vi "Turn On Change Flag Upstream.vi"(8 "symbol to change":T2, 9 "refresh listbox":T1[](array[typedef])) -> (1 "refresh listbox out":T1[](array[typedef]))   [LabVIEW 2020, in "AIM ARINC 429 System Explorer.lvlib" / "Implementation.lvlib"]
uses:
  Implementation.lvlib
  Types/Refresh Symbols.ctl
  Types/Refresh Listbox.ctl
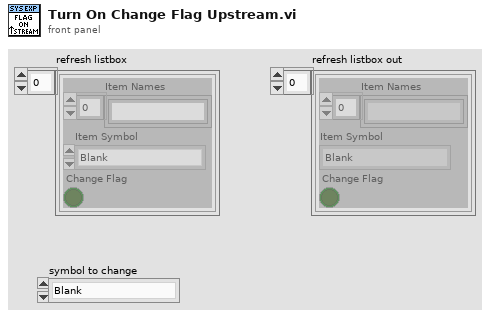
[diagram p1: front panel]
types:
  T1 = typedef "AIM ARINC 429 System Explorer.lvlib/Implementation.lvlib/Refresh Listbox.ctl" = cluster{"Item Names":string[], "Item Symbol":T2, "Change Flag":bool}
  T2 = typedef "AIM ARINC 429 System Explorer.lvlib/Implementation.lvlib/Refresh Symbols.ctl" = enum16{"Blank", "Port", "Incoming", "Outgoing", "Label", "Word", "Parameter", "ARINC-429", "Config Files", "Channel Spec", "Item"}
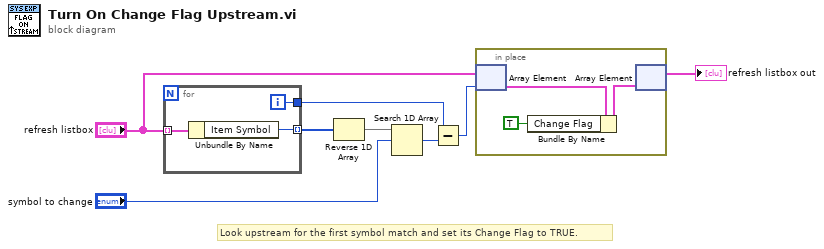
[diagram p0: block diagram]
diagram:
  # "Look upstream for the first symbol match and set its Change Flag to TRUE."
  n1 = for {
    tunnel: "refresh listbox" -> [w11] mode=indexing
    tunnel: [w10] -> w8 mode=indexing
    tunnel: [w9] -> w4
    i -> [w9]
    n2 = Unbundle By Name(w11) -> ("Item Symbol"=w10:T2)
  }
  n3 = Reverse 1D Array(array=w8) -> (reversed array=w7:T2[])
  n4 = Search 1D Array(1D array=w7, element="symbol to change") -> (index of element=w5:i32)  [unwired: 1 in]
  n5 = Subtract(x=w4, y=w5) -> (x-y=w2:i32)
  n6 = in-place {
    n7 = in-place-array #1("refresh listbox", w2) -> (w14:T1)
    n8 = Bundle By Name(cluster=w14, "Change Flag"=TRUE) -> (w13:T1)
    n9 = in-place-array #1(w13) -> (→"refresh listbox out":T1[])  [unwired: 1 out]
  }
